vi "Parse Xml Node Recursively.vi"(7 "Item Data":refnum<class "Item.lvclass">[](array[class]), 8 "error in":errorcluster, 9 "Parents":string[](array[string]), 10 "XML File Path":path, 11 "Node in":refnum<k20>) -> (0 "error out":errorcluster, 3 "Node out":refnum<k20>, 5 "Item Data out":refnum<class "Item.lvclass">[](array[class]))   [LabVIEW 2020, in "VI Properties Editor.lvlib"]
doc: "Parses the XML node recursively, adding more items to <B>Item Data</B>."
uses:
  VI Properties Editor.lvlib
  CTLs/XPath Get Attribute.ctl
  Classes/Item/Item.lvclass
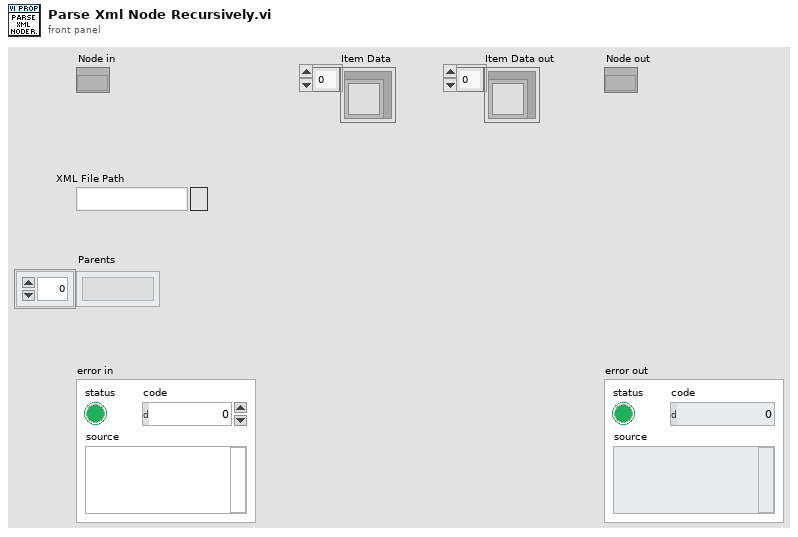
[diagram p1: front panel]
types:
  T1 = typedef "VI Properties Editor.lvlib/XPath Get Attribute.ctl" = enum16{"Item[@Type='VI']/@URL", "Item[@Type='LVClass']/@URL", "Item[@Type='Library']/@URL", "Item[@Type='Folder' and not (@URL)]/@Name", "@Name"}
  T2 = cluster{"XML File Path":path, T1, "Attribute":string[]}
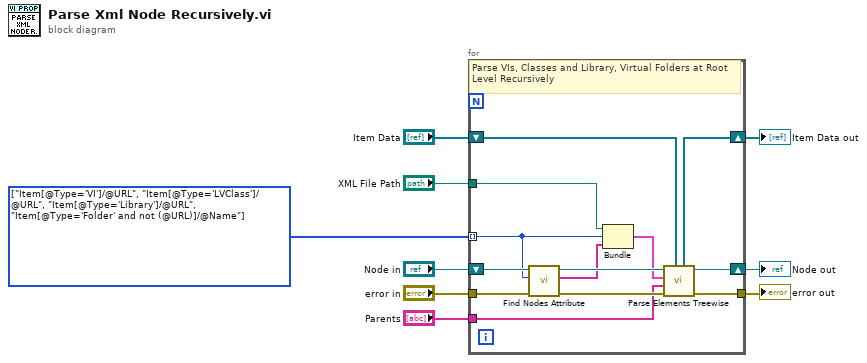
[diagram p0: block diagram]
diagram:
  w7 = T1[] [enum."Item[@Type='VI']/@URL", enum."Item[@Type='LVClass']/@URL", enum."Item[@Type='Library']/@URL", enum."Item[@Type='Folder' and not (@URL)]/@Name"] items=["Item[@Type='VI']/@URL", "Item[@Type='LVClass']/@URL", "Item[@Type='Library']/@URL", "Item[@Type='Folder' and not (@URL)]/@Name", "@Name"] ("XPath Get Attribute")
  n1 = for {
    tunnel: "XML File Path" -> [w16]
    tunnel: [w22] -> w8
    tunnel: "error in" -> [w20]
    tunnel: "Parents" -> [w10]
    shift-right: [w11] -> w3
    shift-left: "Item Data" -> [w12]
    tunnel: w7 -> [w15] mode=indexing
    shift-right: [w17] -> w1
    shift-left: "Node in" -> [w19]
    # "Parse VIs, Classes and Library, Virtual Folders at Root Level Recursively"
    n2 = call "Find Nodes Attribute.vi"("error in (no error)"=w20, "XPath"=w15, "Node in"=w19) -> ("error out"=w21:errorcluster, "Attribute"=w14:string[], "Node out"=w18:refnum<k20>)  [unwired: 6 in]
    n3 = Bundle("XML File Path"=w16, w15, "Attribute"=w14) -> (w13:T2)  [unwired: 1 in]
    n4 = call "Parse Elements Treewise.vi"("Item Data"=w12, "error in"=w21, "Parents"=w10, "XML Info"=w13, "Node in"=w18) -> ("error out"=w22:errorcluster, "Node out"=w17:refnum<k20>, "Item Data out"=w11:refnum<class "Item.lvclass">[])  [unwired: 4 in]
  }
  "error out" <- w8
  "Item Data out" <- w3
  "Node out" <- w1
